vi "Read Configuration Parameters.vi"(8 "error in (no error)":errorcluster, 10 "refnum":T1, 11 "Motions Configuration in":refnum<class "Motions Configuration.lvclass">) -> (0 "error out":errorcluster, 2 "refnum out":T1, 3 "Motions Configuration out":refnum<class "Motions Configuration.lvclass">)   [LabVIEW 2016, in "Hardware.lvlib" / "Motions.lvlib" / "Motions Configuration.lvclass"]
uses:
  <userlib>/Common Components/Hardware/Abstract System/Motions/Motions Config/Motions Configuration.lvclass
  <vilib>/Utility/config.llb/Config Data RefNum.ctl
  <userlib>/Common Components/Hardware/Abstract System/Motions/Motions Config/Motions Configuration.lvclass/Motions Configuration.ctl
  <userlib>/Common Components/Hardware/Abstract System/Motions/Motions/Motions.lvclass/Motions.ctl
  <userlib>/Common Components/Hardware/Abstract System/Motions/Motions/Motions.lvclass
  <userlib>/Common Components/Hardware/Motor/Motor Config/Motor Configuration.lvclass
  <userlib>/Configuration Dialog Actor/Configuration.lvclass
  <vilib>/Utility/config.llb/NI_LVConfig.lvlib
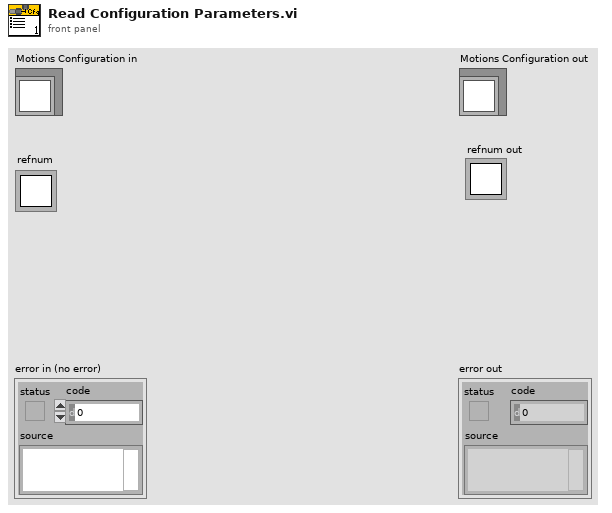
[diagram p1: front panel]
types:
  T1 = typedef "NI_LVConfig.lvlib/Config Data RefNum.ctl" = refnum<k1>
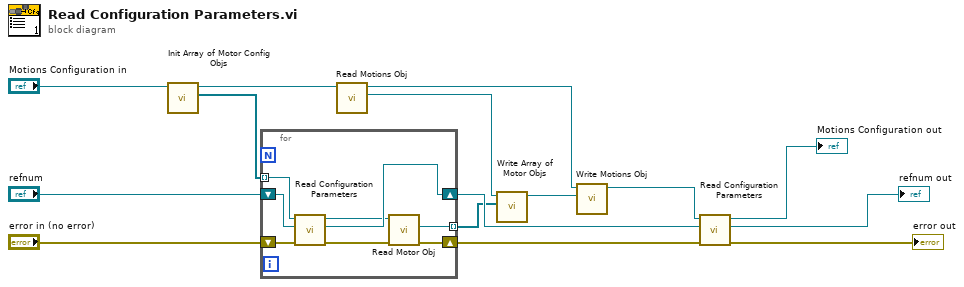
[diagram p0: block diagram]
diagram:
  n1 = call <userlib>:"Init Array of Motor Config Objs.vi"("Motions Configuration in"="Motions Configuration in") -> ("Array of Motor Config Objs"=w10:refnum<class "Motor Configuration.lvclass">[], "Motions Configuration out"=w11:refnum<class "Motions Configuration.lvclass">)  [unwired: 8 in, 1 out]
  n2 = for {
    tunnel: w10 -> [w23] mode=indexing
    shift-right: [w21] -> w6
    shift-left: "refnum" -> [w22]
    shift-right: [w18] -> w7
    shift-left: "error in (no error)" -> [w20]
    tunnel: [w16] -> w1 mode=indexing
    n3 = call-dynamic "Read Configuration Parameters.vi"("error in (no error)"=w20, "refnum"=w22, "Example Configuration Dialog in"=w23) -> ("error out"=w19:errorcluster, "refnum out"=w21:T1, "Example Configuration Dialog out"=w17:refnum<class "Motor Configuration.lvclass">)  [unwired: 6 in]
    n4 = call <userlib>:"Read Motor Obj.vi"("error in (no error)"=w19, "Motor Configuration in"=w17) -> ("error out"=w18:errorcluster, "Hardware.lvlib:Motor.lvlib:Motor.lvclass"=w16:refnum<class "Motor.lvclass">)  [unwired: 7 in, 1 out]
  }
  n5 = call <userlib>:"Read Motions Obj.vi"("Motions Configuration in"=w11) -> ("Hardware.lvlib:Motions.lvlib:Motions.lvclass"=w3:refnum<class "Motions.lvclass">, "Motions Configuration out"=w5:refnum<class "Motions Configuration.lvclass">)  [unwired: 8 in, 1 out]
  n6 = call <userlib>:"Write Array of Motor Objs.vi"("Array of Motor Objs"=w1, "Motions in"=w3) -> ("Motions out"=w2:refnum<class "Motions.lvclass">)  [unwired: 9 in]
  n7 = call <userlib>:"Write Motions Obj.vi"("Hardware.lvlib:Motions.lvlib:Motions.lvclass"=w2, "Motions Configuration in"=w5) -> ("Motions Configuration out"=w4:refnum<class "Motions Configuration.lvclass">)  [unwired: 8 in, 1 out]
  n8 = call-parent "Read Configuration Parameters.vi"("error in (no error)"=w7, "refnum"=w6, "Configuration in"=w4) -> ("error out"=→"error out":errorcluster, "refnum out"=→"refnum out":T1, "Configuration out"=→"Motions Configuration out":refnum<class "Motions Configuration.lvclass">)  [unwired: 6 in]
